vi "Eval Expression String.vi"(8 "error in (no error)":errorcluster, 10 "exprString":string, 11 "PropertyObject in":refnum<class "PropertyObject.lvclass">) -> (0 "error out":errorcluster, 2 "Result":refnum<k7>, 3 "PropertyObject out":refnum<class "PropertyObject.lvclass">)   [LabVIEW 2020, in "TSnax.lvlib" / "PropertyObject.lvclass"]
uses:
  PropertyObject.lvclass
  PropertyObject.lvclass/PropertyObject.ctl
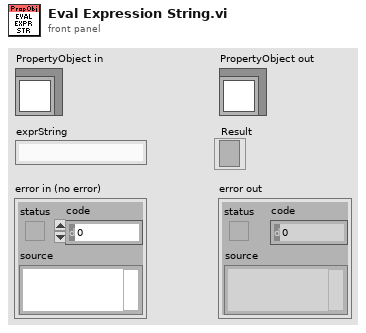
[diagram p1: front panel]
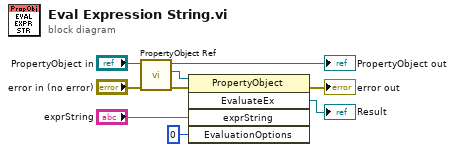
[diagram p0: block diagram]
diagram:
  n1 = call "PropertyObject Ref.vi"("error in (no error)"="error in (no error)", "PropertyObject in"="PropertyObject in") -> ("error out"=w7:errorcluster, "PropertyObject"=w9:refnum<k7>, "PropertyObject out"=→"PropertyObject out":refnum<class "PropertyObject.lvclass">)  [unwired: 7 in]
  n2 = invoke class="PropertyObject" method="EvaluateEx"(reference=w9, error in=w7, "exprString"="exprString", "EvaluationOptions"=0) -> (error out=→"error out":errorcluster, "EvaluateEx"=→"Result":refnum<k7>)  [unwired: 1 in, 3 out]
